vi "Actor Core.vi"(8 "error in":errorcluster, 11 "Measure Object in":refnum<class "Quantum Design.lvclass">) -> (0 "error out":errorcluster, 3 "Actor out":refnum<class "Actor.lvclass">)   [LabVIEW 2018, in "Quantum Design.lvclass"]
doc: "(<B>Filename</B>: Actor Framework.lvlib:Actor.lvclass:Actor Core.vi)\n\nReceives messages to the actor, reacts to them, and initiates any error handling that may shut the actor down.\n\nDescendant classes may override this VI to append parallel tasks for the actor to complete while it handles messages. Overrides use the Call Parent Method node."
uses:
  Quantum Design.lvclass
  <vilib>/ActorFramework/Actor/Actor.lvclass
  NHMFL_Core/Libraries/Instruments/Quantum Design/Quantum Design Driver/Quantum Desing Configuration.ctl
  Instrument Actor/Instrument Actor.lvclass
panel:
  in  "Configuration":T1={"Address"="127.0.0.1", "Instrument type"=0, "Remote"=FALSE, "Measurements"=[enum."Temperature"]} {"Instrument type" items=["PPMS", "VersaLab", "DynaCool", "SVSM"]}
  out "Name":string
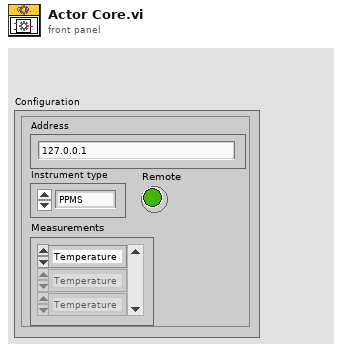
[diagram p1: front panel]
types:
  T1 = typedef "Quantum Desing Configuration.ctl" = cluster{"Address":string, "Instrument type":u16, "Remote":bool, "Measurements":enum16{"Temperature", "Field", "Position"}[]}
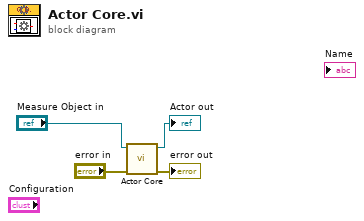
[diagram p0: block diagram]
diagram:
  n1 = call-parent "Actor Core.vi"("error in"="error in", "Measure Object in"="Measure Object in") -> ("error out"=→"error out":errorcluster, "Actor out"=→"Actor out":refnum<class "Actor.lvclass">)  [unwired: 8 in]
